vi "StopVideo.vi"(8 "error in (no error)":errorcluster, 11 "CameraTestingBL in":refnum<class "CameraTesting.lvclass">) -> (0 "error out":errorcluster, 3 "CameraTestingBL out":refnum<class "CameraTesting.lvclass">)   [LabVIEW 2020, in "CameraTesting.lvlib" / "CameraTesting.lvclass"]
doc: "Send command to camera to stopping the data streaming"
uses:
  CameraTesting.lvclass
  CameraTesting.lvclass/CameraTesting.ctl
  Camera/ICamera/ICamera/ICamera.lvclass
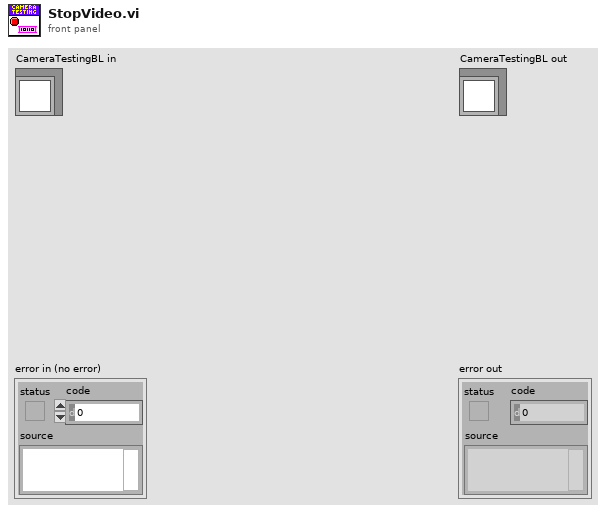
[diagram p1: front panel]
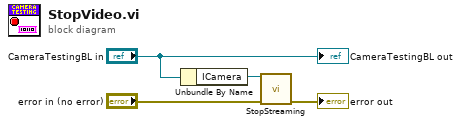
[diagram p0: block diagram]
diagram:
  n1 = Unbundle By Name("CameraTestingBL in") -> ("ICamera"=w3:refnum<class "ICamera.lvclass">)
  n2 = call-dynamic "StopStreaming.vi"("error in (no error)"="error in (no error)", "ICamera in"=w3) -> ("error out"=→"error out":errorcluster)  [unwired: 8 in, 1 out]
  "CameraTestingBL out" <- "CameraTestingBL in"
